vi "automatic_transition.vi"(4 "previous_state":T1, 6 "current_state":T1, 8 "error in (no error)":errorcluster, 10 "index in":i32, 11 "recipe_data in":variant) -> (0 "error out":errorcluster, 2 "index out":i32, 3 "recipe_data out":variant)   [LabVIEW 2015, in "example_01.lvlib"]
uses:
  example_01.lvlib
  lv-recipe-machine/public/_controls/automatic_state.ctl
  lv-recipe-machine/lv-recipe-machine.lvlib
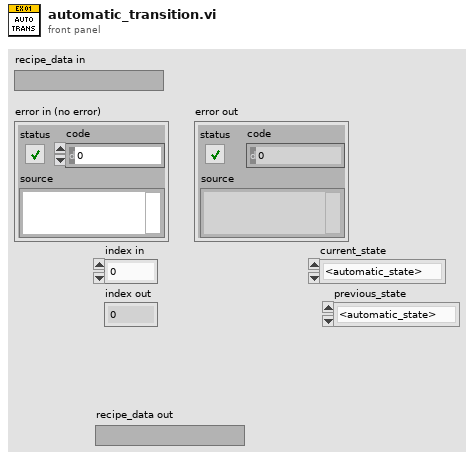
[diagram p1: front panel]
types:
  T1 = typedef "lv-recipe-machine.lvlib/automatic_state.ctl" = enum16{"<automatic_state>", "failed", "idle", "running", "paused", "stopped", "<null>"}
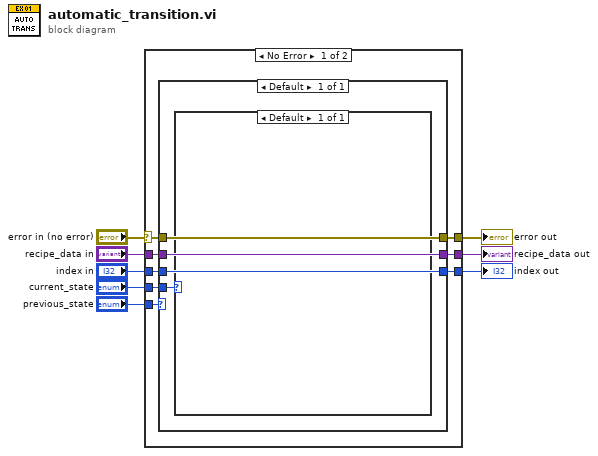
[diagram p0: block diagram]
diagram:
  n1 = case shown="No Error" "error in (no error)" {
    selector: "error in (no error)" -> [w14 w23]
    tunnel: [w13 w23] -> w7
    tunnel: "recipe_data in" -> [w12 w22]
    tunnel: "index in" -> [w10 w21]
    tunnel: "current_state" -> [w15 _]
    tunnel: "previous_state" -> [w16 _]
    tunnel: [w11 w22] -> w2
    tunnel: [w9 w21] -> w1
    frame No Error {
      n2 = case shown="Default" w16 {
        tunnel: w15 -> [w17]
        tunnel: w14 -> [w20]
        tunnel: [w20] -> w13
        tunnel: w12 -> [w19]
        tunnel: [w19] -> w11
        tunnel: w10 -> [w18]
        tunnel: [w18] -> w9
        frame Default {
          n3 = case shown="Default" w17 {
            frame Default {
            }
          }
        }
      }
    }
    frame Error {
    }
  }
  "error out" <- w7
  "recipe_data out" <- w2
  "index out" <- w1
